vi "current version.vi"() -> ()   [LabVIEW 2013, in "Profibus Module configuration.lvclass"]
doc: "#CodeRequired\nThis global variable stores the current version of the module and should be updated as serialization formats change."
uses:
  Profibus Module configuration.lvclass
panel:
  out "current version":string="1.2.0.0"
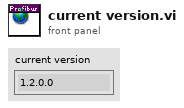
[diagram p1: front panel]
diagram:
